vi "IMAQdx Release Image.vi"(8 "error in":errorcluster, 9 "Buffer Number In":u32, 10 "Image":T1, 11 "Session In":T2) -> (0 "error out":errorcluster, 3 "Session Out":T2)   [LabVIEW 2020, in "NI_Vision_Acquisition_Software.lvlib"]
doc: "Releases the specified extracted image, thus allowing the acquisition to proceed."
uses:
  NI_Vision_Acquisition_Software.lvlib
  IMAQdx.ctl
  IMAQ Image.ctl
  niimaqdx.dll
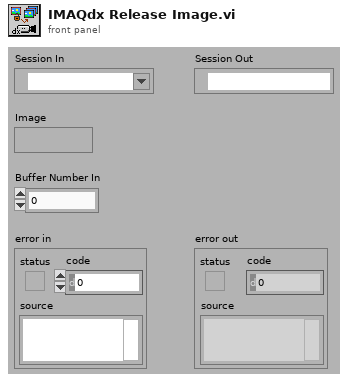
[diagram p1: front panel]
types:
  T1 = typedef "IMAQ Image.ctl" = refnum<image>
  T2 = typedef "IMAQdx.ctl" = refnum<k21>
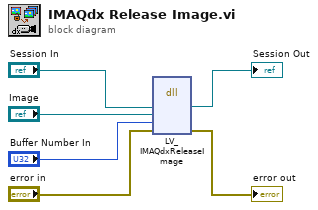
[diagram p0: block diagram]
diagram:
  n1 = dll-call lib="niimaqdx.dll" fn="LV_IMAQdxReleaseImage"("refnum"="Session In", "image"="Image", "bufferNumber"="Buffer Number In", "error"="error in") -> ("refnum"=→"Session Out":T2, "error"=→"error out":errorcluster)  [unwired: 6 in, 2 out]
